vi "GetVariable.vi"(8 "error in":errorcluster, 9 "variable":string, 11 "lua_State *L":u64) -> (0 "error out":errorcluster, 3 "value":dbl)   [LabVIEW 2011]
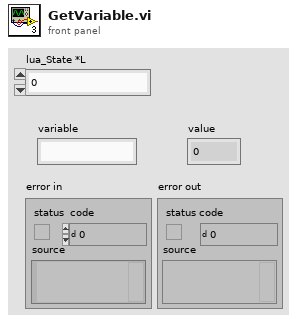
[diagram p1: front panel]
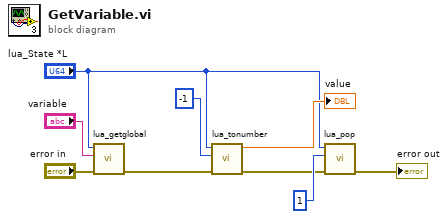
[diagram p0: block diagram]
diagram:
  n1 = call "lua_getglobal.vi"("error in"="error in", "const char *name"="variable", "lua_State *L"="lua_State *L") -> ("error out"=w6:errorcluster)  [unwired: 8 in]
  n2 = call "lua_tonumber.vi"("error in"=w6, "index"=-1, "lua_State *L"="lua_State *L") -> ("error out"=w2:errorcluster, "lua_Number"=→"value":dbl)  [unwired: 7 in]
  n3 = call "lua_pop.vi"("error in"=w2, "n"=1, "lua_State *L"="lua_State *L") -> ("error out"=→"error out":errorcluster)  [unwired: 8 in]
